vi "main.vi"() -> ()   [LabVIEW 2016]
uses:
  enum_setting_states.ctl
  <vilib>/Instr/_visa.llb/VISA Configure Serial Port (Instr).vi
  global.vi
panel:
  out "Tab Control":enum32{"Settings", "Data"}(tab)
  in  "Boolean":bool
  in  "4th":dbl=4.0 min=1.0 step=1.0 format="%#_3g"
  in  "3rd":dbl=3.0 min=1.0 step=1.0 format="%#_3g"
  in  "2nd":dbl=2.0 min=1.0 step=1.0 format="%#_3g"
  in  "1st":dbl=1.0 min=1.0 step=1.0 format="%#_3g"
  in  "START":bool
  in  "SET":bool
  in  "Flow control (None)":u16(ring) items=["None", "XON/XOFF", "RTS/CTS", "XON/XOFF & RTS/CTS", "DTR/DSR", "XON/XOFF & DTR/DSR"]
  in  "Parity (None)":enum16{"None", "Odd", "Even", "Mark", "Space"}(ring)
  in  "Stop bits (1)":u16(ring)=10 items=["1.0"=10, "1.5"=15, "2.0"=20]
  in  "Data bits (8)":u16=8 min=5 max=8 step=1
  in  "Baud rate":u32=57600
  in  "VISA resource name":refnum<visa-resource-name>="COM5"
  out "read buffer":string
  in  "Charge current":enum8{"0.25C", "0.5C", "1C"}(ring)=enum."0.5C"
  in  "Discharge current":enum8{"0.25C", "0.5C", "1C"}(ring)=enum."1C"
  in  "Number of cells":enum8{"", "1", "2", "3", "4"}(ring)=enum."1"
  in  "Options":T1(ring)=enum."Predischarge->Charge->Discharge->Postcharge"
  in  "Project Name":string="Test"
  out "Cell number":string
  out "State":string
  out "Path":path
  in  "stop":bool
  out "TEMP":dbl caption="Current Temperature\n(Celsius)"
  out "CURRENT":dbl caption="Current Temperature\n(Celsius)"
  out "VOLTAGE":dbl caption="Current Temperature\n(Celsius)"
  in  "next":bool
  out "Countdown":dbl caption="Current Temperature\n(Celsius)"
  out "min":dbl caption="Current Temperature\n(Celsius)"
  out "sec":dbl caption="Current Temperature\n(Celsius)"
  out "CAPACITY":dbl caption="Current Temperature\n(Celsius)"
  out "Voltage":cluster{dbl[], dbl[]}(graph)
  out "Current":cluster{dbl[], dbl[]}(graph)
  out "Temperature":cluster{dbl[], dbl[]}(graph)
  out "Capacity":cluster{dbl[], dbl[]}(graph)
  out "Received data":string
  # "UART configurations"
  # "Test configurations"
  # "Cell order"
  # "Elapsed time"
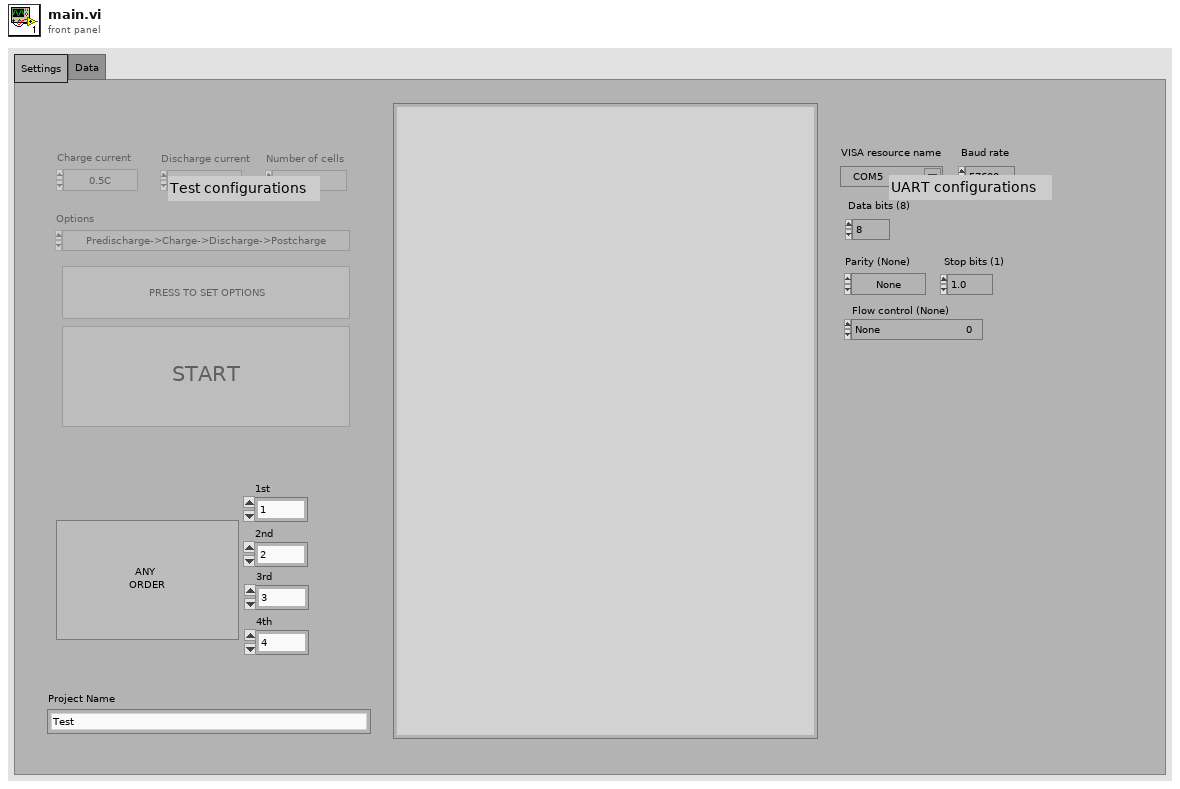
[diagram p1: front panel]
types:
  T1 = enum8{"", "Predischarge->Charge->Discharge->Postcharge", "Charge->Discharge", "Only Charge", "Only Discharge"}
  T2 = enum8{"Enabled", "Disabled", "Disabled and Grayed Out"}
  T3 = typedef "enum_setting_states.ctl" = enum16{"Initialize", "Charge_current", "Discharge_current", "Option", "Num_of_cells", "Start"}
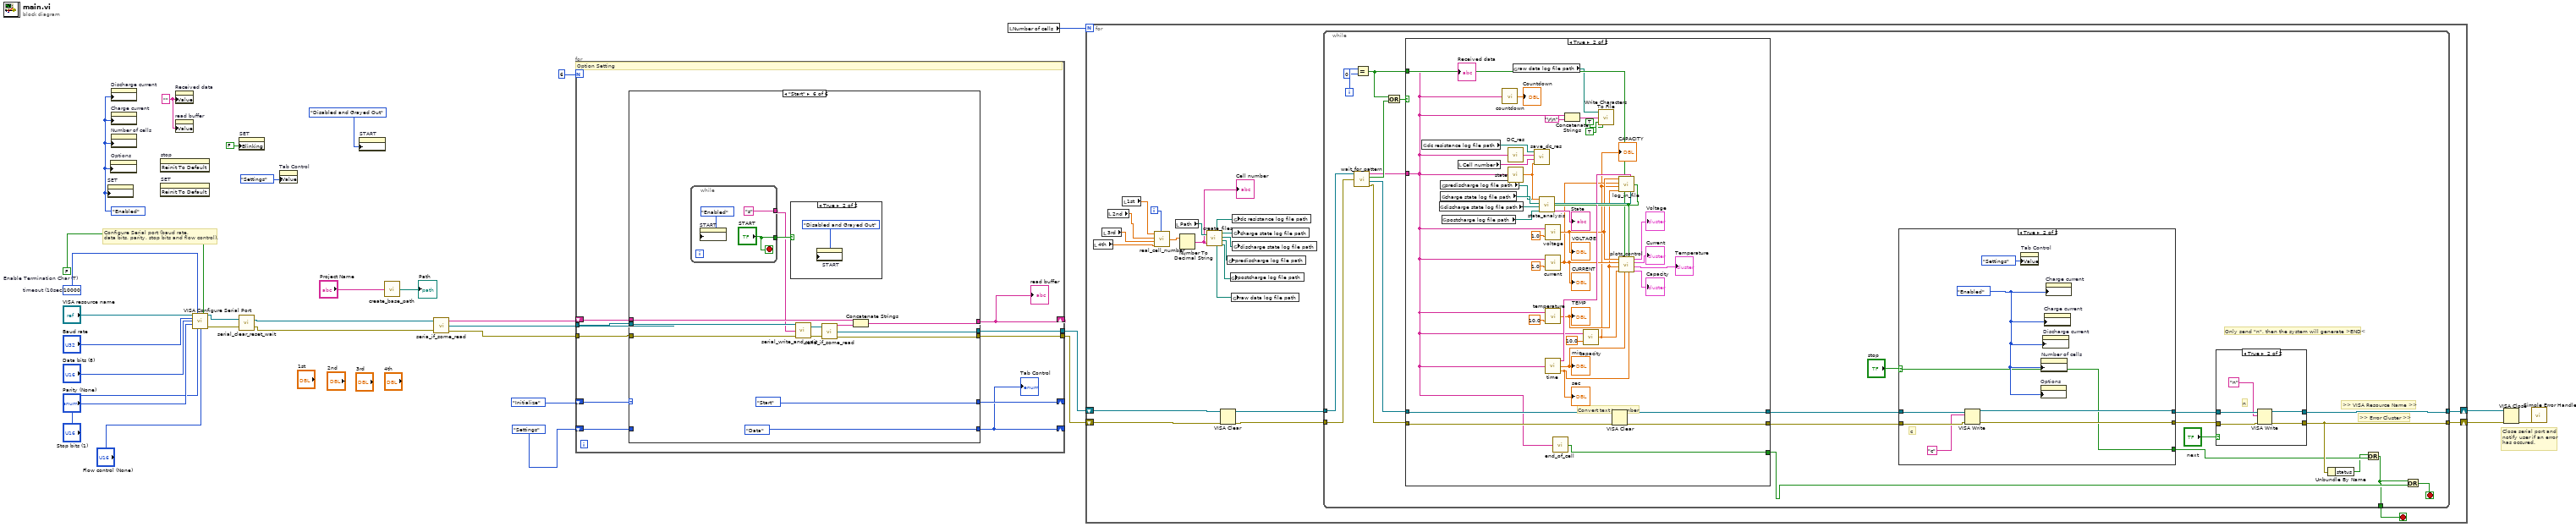
[diagram p0: block diagram]
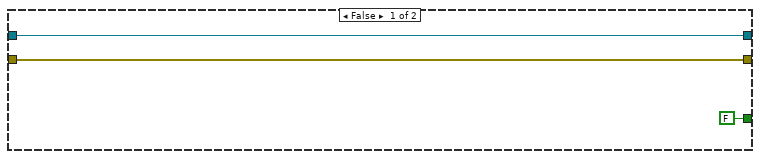
[diagram p2: hidden frame]
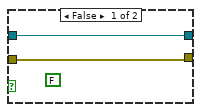
[diagram p3: hidden frame]
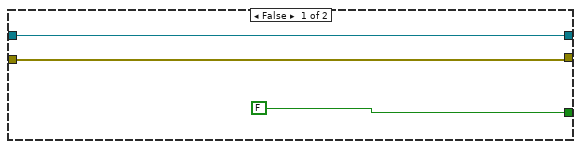
[diagram p4: hidden frame]
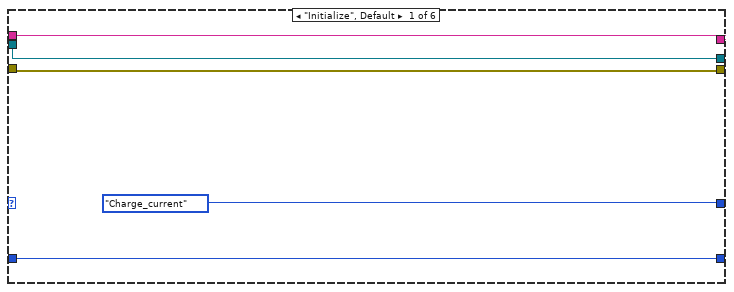
[diagram p5: hidden frame]
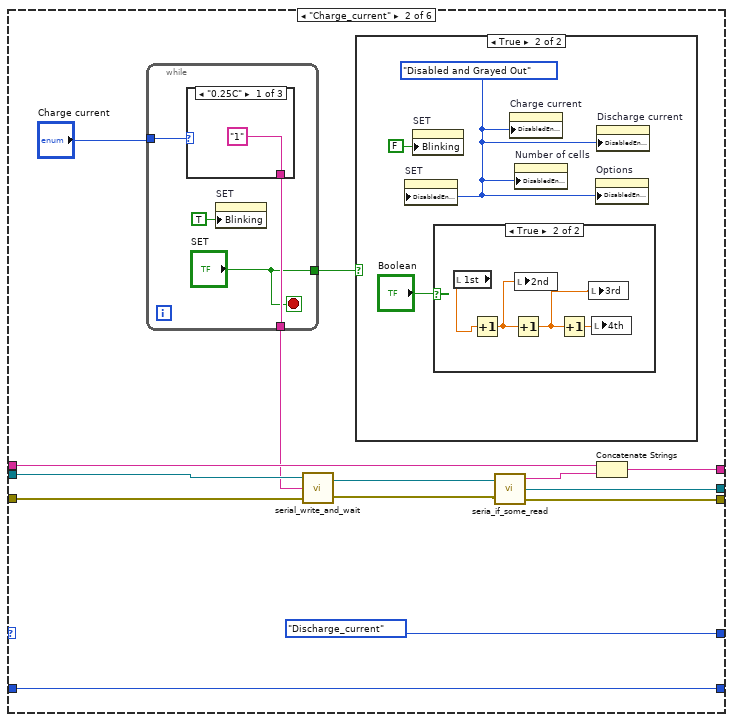
[diagram p6: hidden frame]
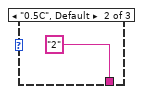
[diagram p9: hidden frame]
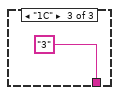
[diagram p10: hidden frame]
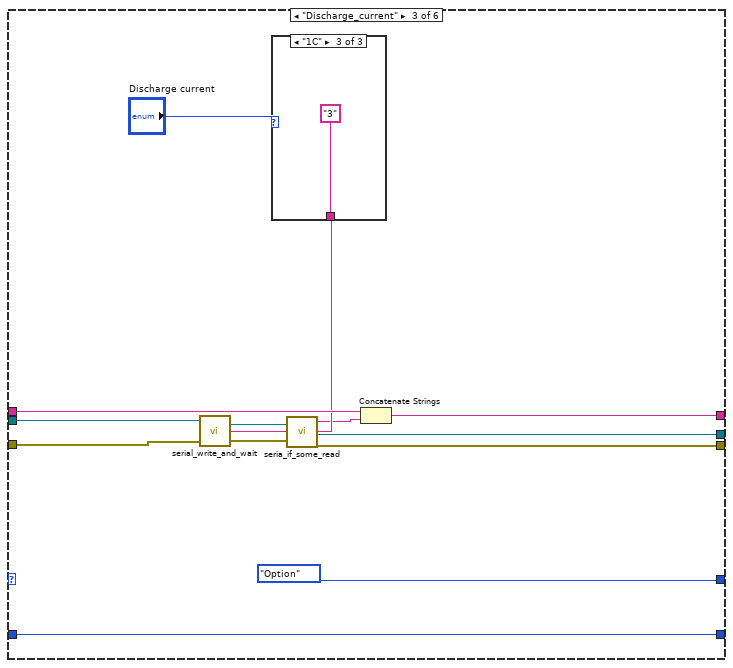
[diagram p11: hidden frame]
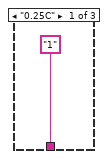
[diagram p12: hidden frame]
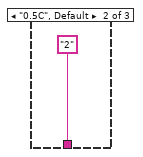
[diagram p13: hidden frame]
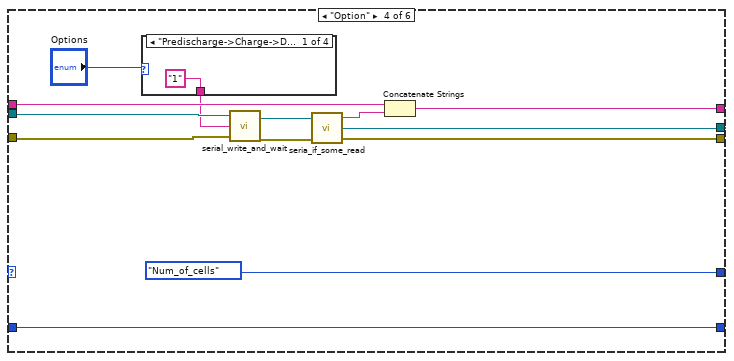
[diagram p14: hidden frame]
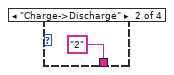
[diagram p15: hidden frame]
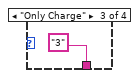
[diagram p16: hidden frame]
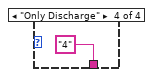
[diagram p17: hidden frame]
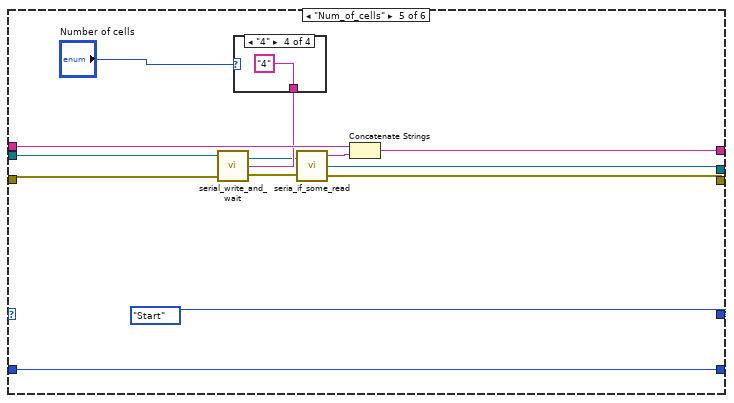
[diagram p18: hidden frame]
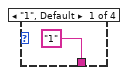
[diagram p19: hidden frame]
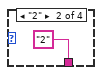
[diagram p20: hidden frame]
diagram:
  w11 = T2."Enabled" ("Disabled")
  w9 = "" ("read buffer")
  w30 = FALSE  # Enable Termination Char (T)
  w31 = u32 10000  # timeout (10sec)
  # "Close serial port and\nnotify user if an error\nhas occured."
  # "Configure Serial port (baud rate,\ndata bits, parity, stop bits and flow control)."
  n1 = property on="SET" class="Bool (strict)"("DisabledEnum"=w11) -> ()  [unwired: 2 in, 2 out]
  n2 = property on="Options" class="Enum (strict)"("DisabledEnum"=w11) -> ()  [unwired: 2 in, 2 out]
  n3 = property on="Discharge current" class="Enum (strict)"("DisabledEnum"=w11) -> ()  [unwired: 2 in, 2 out]
  n4 = property on="Charge current" class="Enum (strict)"("DisabledEnum"=w11) -> ()  [unwired: 2 in, 2 out]
  n5 = property on="Number of cells" class="Enum (strict)"("DisabledEnum"=w11) -> ()  [unwired: 2 in, 2 out]
  n6 = invoke on="stop" class="Bool" method="Reinit To Default"() -> ()  [unwired: 3 in, 3 out]
  n7 = invoke on="SET" class="Bool (strict)" method="Reinit To Default"() -> ()  [unwired: 3 in, 3 out]
  n8 = property on="Received data" class="Str"("Value"=w9) -> ()  [unwired: 2 in, 2 out]
  n9 = property on="read buffer" class="Str"("Value"=w9) -> ()  [unwired: 2 in, 2 out]
  n10 = call-poly "VISA Configure Serial Port"("VISA resource name"="VISA resource name", "timeout (10sec)"=w31, "Enable Termination\nChar (T)"=w30, "baud rate (9600)"="Baud rate", "data bits (8)"="Data bits (8)", "parity (0:none)"="Parity (None)", "stop bits (10: 1 bit)"="Stop bits (1)", "flow control (0:none)"="Flow control (None)") -> ("VISA resource name out"=w28:refnum<visa-resource-name>, "error out"=w29:errorcluster)  [unwired: 6 in]
  n11 = property on="SET" class="Bool (strict)"("Blinking"=FALSE) -> ()  [unwired: 2 in, 2 out]
  n12 = call "serial_clear_reset_wait.vi"("error in (no error)"=w29, "VISA Refnum in"=w28) -> ("error out"=w14:errorcluster, "VISA Refnum out"=w15:refnum<visa-resource-name>)
  n13 = property on="Tab Control" class="TabCtl (strict)"("Value"=enum32{"Settings", "Data"}."Settings" ("Tab Control")) -> ()  [unwired: 2 in, 2 out]
  n14 = property on="START" class="Bool"("DisabledEnum"=T2."Disabled and Grayed Out" ("Disabled")) -> ()  [unwired: 2 in, 2 out]
  n15 = call "create_base_path.vi"("project name"="Project Name") -> ("base path"=→"Path":path)
  n16 = call "seria_if_some_read.vi"("serial in"=w15, "error in (no error)"=w14) -> ("read buffer"=w7:string, "serial out"=w8:refnum<visa-resource-name>, "error out"=w16:errorcluster)
  n17 = for {
    N: 6 -> [_]
    shift-right: [w32] -> _
    shift-left: enum32{"Settings", "Data"}."Settings" ("Tab Control") -> [w39]
    shift-right: [w38] -> _
    shift-left: enum_setting_states."Initialize" -> [w37]
    tunnel: w8 -> [w35]
    tunnel: [w41] -> w3
    tunnel: w16 -> [w34]
    tunnel: [w40] -> w2
    shift-right: [w36] -> _
    shift-left: w7 -> [w33]
    # "Option Setting"
    n18 = case shown="\"Start\"" w37 {
      tunnel: w35 -> [w45 w59 w83 w96 w116 w132]
      tunnel: w34 -> [w44 w58 w81 w94 w114 w131]
      tunnel: [w43 w56 w85 w102 w118 w137] -> w36
      tunnel: [w45 w49 w77 w98 w110 w126] -> w41
      tunnel: [w44 w48 w76 w97 w109 w125] -> w40
      tunnel: [w42 w53 w84 w100 w117 enum32{"Settings", "Data"}."Data" ("Tab Control")] -> w32
      tunnel: w39 -> [w42 w53 w84 w100 w117 _]
      tunnel: [enum_setting_states."Charge_current" enum_setting_states."Discharge_current" enum_setting_states."Option" enum_setting_states."Num_of_cells" enum_setting_states."Start" enum_setting_states."Start"] -> w38
      tunnel: w33 -> [w43 w57 w86 w103 w119 w136]
      frame "Initialize", Default {
      }
      frame "Charge_current" {
        n19 = while {
          tunnel: "Charge current" -> [w71]
          tunnel: [w70] -> w55
          tunnel: ["SET"] -> w54
          stop <- "SET" stop-if-true
          n20 = case shown="\"0.25C\"" w71 {
            tunnel: ["1" ("write buffer") "2" ("write buffer") "3" ("write buffer")] -> w70
            frame "0.25C" {
            }
            frame "0.5C", Default {
            }
            frame "1C" {
            }
          }
          n21 = property on="SET" class="Bool (strict)"("Blinking"=TRUE) -> ()  [unwired: 2 in, 2 out]
        }
        n22 = call "serial_write_and_wait.vi"("error in (no error)"=w58, "write buffer"=w55, "serial in"=w59) -> ("error out"=w51:errorcluster, "serial out"=w52:refnum<visa-resource-name>)
        n23 = case shown="True" w54 {
          frame False {
          }
          frame True {
            w62 = T2."Disabled and Grayed Out" ("Disabled")
            n24 = property on="SET" class="Bool (strict)"("DisabledEnum"=w62) -> ()  [unwired: 2 in, 2 out]
            n25 = property on="SET" class="Bool (strict)"("Blinking"=FALSE) -> ()  [unwired: 2 in, 2 out]
            n26 = case shown="True" "Boolean" {
              frame False {
              }
              frame True {
                n27 = local read "1st"() -> (w66:dbl)
                n28 = Increment(x=w66) -> (x+1=w67:dbl)
                n29 = Increment(x=w67) -> (x+1=w64:dbl)
                n30 = local write "2nd"(w67) -> ()
                n31 = Increment(x=w64) -> (x+1=w65:dbl)
                n32 = local write "3rd"(w64) -> ()
                n33 = local write "4th"(w65) -> ()
              }
            }
            n34 = property on="Charge current" class="Enum (strict)"("DisabledEnum"=w62) -> ()  [unwired: 2 in, 2 out]
            n35 = property on="Number of cells" class="Enum (strict)"("DisabledEnum"=w62) -> ()  [unwired: 2 in, 2 out]
            n36 = property on="Options" class="Enum (strict)"("DisabledEnum"=w62) -> ()  [unwired: 2 in, 2 out]
            n37 = property on="Discharge current" class="Enum (strict)"("DisabledEnum"=w62) -> ()  [unwired: 2 in, 2 out]
          }
        }
        n38 = call "seria_if_some_read.vi"("serial in"=w52, "error in (no error)"=w51) -> ("read buffer"=w50:string, "serial out"=w49:refnum<visa-resource-name>, "error out"=w48:errorcluster)
        n39 = Concatenate Strings(w57, w50) -> (w56:string)
      }
      frame "Discharge_current" {
        n40 = case shown="\"1C\"" "Discharge current" {
          tunnel: ["1" ("write buffer") "2" ("write buffer") "3" ("write buffer")] -> w82
          frame "0.25C" {
          }
          frame "0.5C", Default {
          }
          frame "1C" {
          }
        }
        n41 = call "serial_write_and_wait.vi"("error in (no error)"=w81, "write buffer"=w82, "serial in"=w83) -> ("error out"=w79:errorcluster, "serial out"=w80:refnum<visa-resource-name>)
        n42 = call "seria_if_some_read.vi"("serial in"=w80, "error in (no error)"=w79) -> ("read buffer"=w78:string, "serial out"=w77:refnum<visa-resource-name>, "error out"=w76:errorcluster)
        n43 = Concatenate Strings(w86, w78) -> (w85:string)
      }
      frame "Option" {
        n44 = case shown="\"Predischarge->Charge->Discharge->Postcharge\", Default" "Options" {
          tunnel: ["1" ("write buffer") "2" ("write buffer") "3" ("write buffer") "4" ("write buffer")] -> w95
          frame "Predischarge->Charge->Discharge->Postcharge", Default {
          }
          frame "Charge->Discharge" {
          }
          frame "Only Charge" {
          }
          frame "Only Discharge" {
          }
        }
        n45 = call "serial_write_and_wait.vi"("error in (no error)"=w94, "write buffer"=w95, "serial in"=w96) -> ("error out"=w92:errorcluster, "serial out"=w93:refnum<visa-resource-name>)
        n46 = call "seria_if_some_read.vi"("serial in"=w93, "error in (no error)"=w92) -> ("read buffer"=w99:string, "serial out"=w98:refnum<visa-resource-name>, "error out"=w97:errorcluster)
        n47 = Concatenate Strings(w103, w99) -> (w102:string)
      }
      frame "Num_of_cells" {
        n48 = case shown="\"4\"" "Number of cells" {
          tunnel: ["1" ("write buffer") "2" ("write buffer") "3" ("write buffer") "4" ("write buffer")] -> w115
          frame "1", Default {
          }
          frame "2" {
          }
          frame "3" {
          }
          frame "4" {
          }
        }
        n49 = call "serial_write_and_wait.vi"("error in (no error)"=w114, "write buffer"=w115, "serial in"=w116) -> ("error out"=w112:errorcluster, "serial out"=w113:refnum<visa-resource-name>)
        n50 = call "seria_if_some_read.vi"("serial in"=w113, "error in (no error)"=w112) -> ("read buffer"=w111:string, "serial out"=w110:refnum<visa-resource-name>, "error out"=w109:errorcluster)
        n51 = Concatenate Strings(w119, w111) -> (w118:string)
      }
      frame "Start" {
        n52 = while {
          tunnel: ["s" ("write buffer")] -> w130
          tunnel: ["START"] -> w133
          stop <- "START" stop-if-true
          n53 = property on="START" class="Bool"("DisabledEnum"=T2."Enabled" ("Disabled")) -> ()  [unwired: 2 in, 2 out]
        }
        n54 = case shown="True" w133 {
          frame False {
          }
          frame True {
            n55 = property on="START" class="Bool"("DisabledEnum"=T2."Disabled and Grayed Out" ("Disabled")) -> ()  [unwired: 2 in, 2 out]
          }
        }
        n56 = call "serial_write_and_wait.vi"("error in (no error)"=w131, "write buffer"=w130, "serial in"=w132) -> ("error out"=w128:errorcluster, "serial out"=w129:refnum<visa-resource-name>)
        n57 = call "seria_if_some_read.vi"("serial in"=w129, "error in (no error)"=w128) -> ("read buffer"=w127:string, "serial out"=w126:refnum<visa-resource-name>, "error out"=w125:errorcluster)
        n58 = Concatenate Strings(w136, w127) -> (w137:string)
      }
    }
    "read buffer" <- w36
    "Tab Control" <- w32
  }
  n59 = local read "Number of cells"() -> (w1:enum8{"", "1", "2", "3", "4"})
  n60 = for {
    N: w1 -> [_]
    shift-right: [w160] -> w20
    shift-left: w3 -> [w158]
    shift-right: [w159] -> w19
    shift-left: w2 -> [w157]
    i -> [w145]
    stop <- w142 stop-if-true
    n61 = local read "4th"() -> (w156:dbl)
    n62 = local read "3rd"() -> (w155:dbl)
    n63 = local read "2nd"() -> (w154:dbl)
    n64 = local read "1st"() -> (w153:dbl)
    n65 = call "real_cell_number.vi"("1st"=w153, "2nd"=w154, "3rd"=w155, "4th"=w156, "current loop (cell)"=w145) -> ("real cell number"=w152:dbl)
    n66 = local read "Path"() -> (w151:path)
    n67 = Number To Decimal String(number=w152) -> (decimal integer string=w146:string)  [unwired: 1 in]
    "Cell number" <- w146
    n68 = call "create_files.vi"("base path"=w151, "cell number string"=w146) -> ("dc resistance log file path"=w147:path, "raw data log file path"=w150:path, "charge state log file path"=w149:path, "discharge state log file path"=w148:path, "predischarge state log file path"=w144:path, "postcharge state log file path"=w143:path)
    n69 = VISA Clear(VISA resource name=w158, error in (no error)=w157) -> (VISA resource name out=w162:refnum<visa-resource-name>, error out=w161:errorcluster)
    n70 = global write "global.vi" "predischarge log file path"(w144) -> ()
    n71 = global write "global.vi" "postcharge log file path"(w143) -> ()
    n72 = global write "global.vi" "raw data log file path"(w150) -> ()
    n73 = global write "global.vi" "dc resistance log file path"(w147) -> ()
    n74 = global write "global.vi" "charge state log file path"(w149) -> ()
    n75 = global write "global.vi" "discharge state log file path"(w148) -> ()
    n76 = while {
      tunnel: [w182] -> w160
      tunnel: w162 -> [w173]
      tunnel: w161 -> [w172]
      tunnel: [w181] -> w159
      tunnel: [w163] -> w142
      i -> [w178]
      stop <- w165 stop-if-true
      # "Only send \"n\", then the system will generate >END<"
      # ">> Error Cluster >>"
      # ">> VISA Resource Name >>"
      n77 = call "wait_for_pattern.vi"("serial in"=w173, "error in (no error)"=w172) -> ("pattern string"=w168:string, "pattern detected"=w171:bool, "serial out"=w169:refnum<visa-resource-name>, "error out"=w170:errorcluster)  [unwired: 1 in]
      n78 = Equal?(x=w178, y=0) -> (x = y?=w175:bool)
      n79 = Or(x=w175, y=w171) -> (x .or. y?=w176:bool)
      n80 = case shown="True" w176 {
        tunnel: w168 -> [_ w190]
        tunnel: w169 -> [w188 w209]
        tunnel: w170 -> [w187 w207]
        tunnel: [w187 w206] -> w180
        tunnel: [w188 w208] -> w179
        tunnel: w175 -> [_ w198]
        tunnel: [FALSE ("Boolean") w189] -> w164
        frame False {
        }
        frame True {
          # "Convert text to number"
          n81 = global read "global.vi" "dc resistance log file path"() -> (w194:path)
          n82 = global read "global.vi" "discharge state log file path"() -> (w196:path)
          n83 = global read "global.vi" "predischarge log file path"() -> (w195:path)
          n84 = global read "global.vi" "charge state log file path"() -> (w197:path)
          n85 = global read "global.vi" "postcharge log file path"() -> (w191:path)
          n86 = local read "Cell number"() -> (w192:string)
          n87 = call "countdown.vi"("buffer in"=w190) -> ("countdown"=→"Countdown":dbl)
          n88 = call "DC_res.vi"("read buffer in"=w190) -> ("read buffer out"=w220:string)
          n89 = call "state.vi"("buffer in"=w190) -> ("current state"=w219:dbl)
          n90 = global read "global.vi" "raw data log file path"() -> (w193:path)
          n91 = call "save_dc_res.vi"("current state"=w219, "cell number"=w192, "dc resistance"=w220, "file path"=w194) -> ()
          n92 = call "state_analysis.vi"("current state number"=w219, "postcharge state log file path"=w191, "discharge state log file path"=w196, "charge state log file path"=w197, "predischarge state log file path"=w195) -> ("current state name"=→"State":string, "log? plot?"=w205:bool, "chosen log file path"=w223:path)
          n93 = call "time.vi"("buffer in"=w190) -> ("mm:ss"=w218:string, "minutes"=w204:dbl, "seconds"=w203:dbl)
          "min" <- w204
          "sec" <- w203
          n94 = call "voltage.vi"("divider"=1.0 ("y"), "buffer in"=w190) -> ("voltage"=w202:dbl)
          "VOLTAGE" <- w202
          n95 = call "current.vi"("divider"=1.0 ("y"), "buffer in"=w190) -> ("current"=w201:dbl)
          "CURRENT" <- w201
          n96 = call "temperature.vi"("divider"=10.0 ("y"), "buffer in"=w190) -> ("temperature"=w200:dbl)
          "TEMP" <- w200
          n97 = call "end_of_cell.vi"("buffer in"=w190) -> ("Boolean"=w189:bool)
          n98 = Concatenate Strings(w190, "\r\n") -> (w213:string)
          n99 = call "capacity.vi"("divider"=10.0 ("y"), "buffer in"=w190) -> ("capacity"=w199:dbl)
          "CAPACITY" <- w199
          n100 = call <vilib>:"Write Characters To File.vi"("convert eol? (no:F)"=TRUE, "append to file? (new file:F)"=TRUE, "character string"=w213, "file path (dialog if empty)"=w193) -> ()  [unwired: 1 in, 1 out]
          n101 = VISA Clear(VISA resource name=w209, error in (no error)=w207) -> (VISA resource name out=w208:refnum<visa-resource-name>, error out=w206:errorcluster)
          n102 = call "log_in_file.vi"("file path"=w223, "save?"=w205, "mm:ss"=w218, "temperature"=w200, "capacity"=w199, "current"=w201, "voltage"=w202) -> ()
          n103 = call "plots_control.vi"("seconds"=w203, "log? plot?"=w205, "minutes"=w204, "is first loop?"=w198, "capacity"=w199, "temperature"=w200, "current"=w201, "voltage"=w202) -> ("capacity cluster"=→"Capacity":cluster{dbl[], dbl[]}, "temperature cluster"=→"Temperature":cluster{dbl[], dbl[]}, "current cluster"=→"Current":cluster{dbl[], dbl[]}, "voltage cluster"=→"Voltage":cluster{dbl[], dbl[]})
          "Received data" <- w190
        }
      }
      n104 = case shown="True" "stop" {
        selector: "stop" -> [_ w239]
        tunnel: w179 -> [w236 w245]
        tunnel: [w236 w244] -> w184
        tunnel: w180 -> [w237 w243]
        tunnel: [w237 w242] -> w183
        tunnel: [FALSE w239] -> w167
        frame False {
        }
        frame True {
          w240 = T2."Enabled" ("Disabled")
          # "c"
          n105 = VISA Write(VISA resource name=w245, write buffer="c", error in (no error)=w243) -> (VISA resource name out=w244:refnum<visa-resource-name>, error out=w242:errorcluster)  [unwired: 1 out]
          n106 = property on="Tab Control" class="TabCtl (strict)"("Value"=enum32{"Settings", "Data"}."Settings" ("Tab Control")) -> ()  [unwired: 2 in, 2 out]
          n107 = property on="Options" class="Enum (strict)"("DisabledEnum"=w240) -> ()  [unwired: 2 in, 2 out]
          n108 = property on="Number of cells" class="Enum (strict)"("DisabledEnum"=w240) -> ()  [unwired: 2 in, 2 out]
          n109 = property on="Discharge current" class="Enum (strict)"("DisabledEnum"=w240) -> ()  [unwired: 2 in, 2 out]
          n110 = property on="Charge current" class="Enum (strict)"("DisabledEnum"=w240) -> ()  [unwired: 2 in, 2 out]
          n111 = property on="Charge current" class="Enum (strict)"("DisabledEnum"=w240) -> ()  [unwired: 2 in, 2 out]
        }
      }
      n112 = case shown="True" "next" {
        tunnel: w184 -> [w228 w234]
        tunnel: [w228 w233] -> w182
        tunnel: w183 -> [w229 w232]
        tunnel: [w229 w231] -> w181
        frame False {
          (unwired) FALSE
        }
        frame True {
          # "n"
          n113 = VISA Write(VISA resource name=w234, write buffer="n", error in (no error)=w232) -> (VISA resource name out=w233:refnum<visa-resource-name>, error out=w231:errorcluster)  [unwired: 1 out]
        }
      }
      n114 = Unbundle By Name(w181) -> ("status"=w166:bool)
      n115 = Or(x=w166, y=w167) -> (x .or. y?=w163:bool)
      n116 = Or(x=w163, y=w164) -> (x .or. y?=w165:bool)
    }
  }
  n117 = VISA Close(VISA resource name=w20, error in (no error)=w19) -> (error out=w21:errorcluster)
  n118 = call <vilib>:"Simple Error Handler.vi"("error in (no error)"=w21) -> ()  [unwired: 4 in, 5 out]
